vi "__AttrMap-SetValue2.vi"(8 "error in (no error)":errorcluster, 9 "Key":string, 10 "Value":variant, 11 "AttrMap in":T1) -> (0 "error out":errorcluster, 3 "AttrMap out":T1)   [LabVIEW 2019]
uses:
  Typedef/Def-AttrMap.ctl
  6e91e2cf-a420-477d-bf86-627245081caf.vi
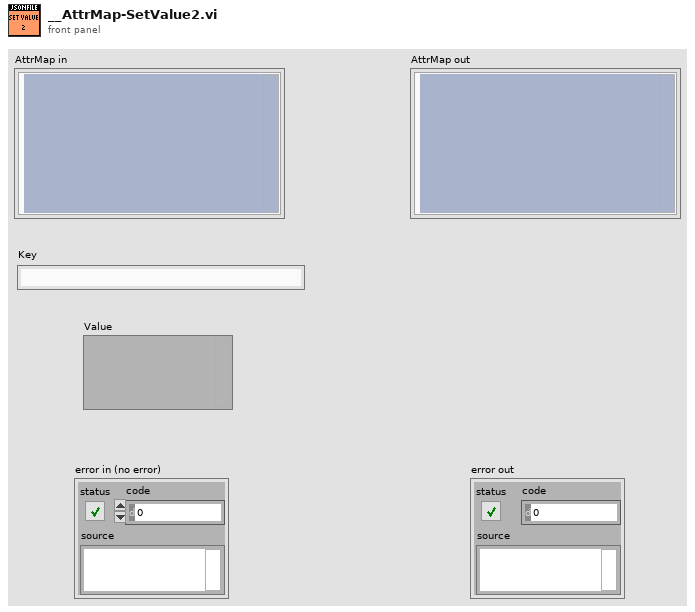
[diagram p1: front panel]
types:
  T1 = typedef "Def-AttrMap.ctl" = cluster{"Map":variant}
  T2 = typedef "Def-NameMap.ctl" = variant[]
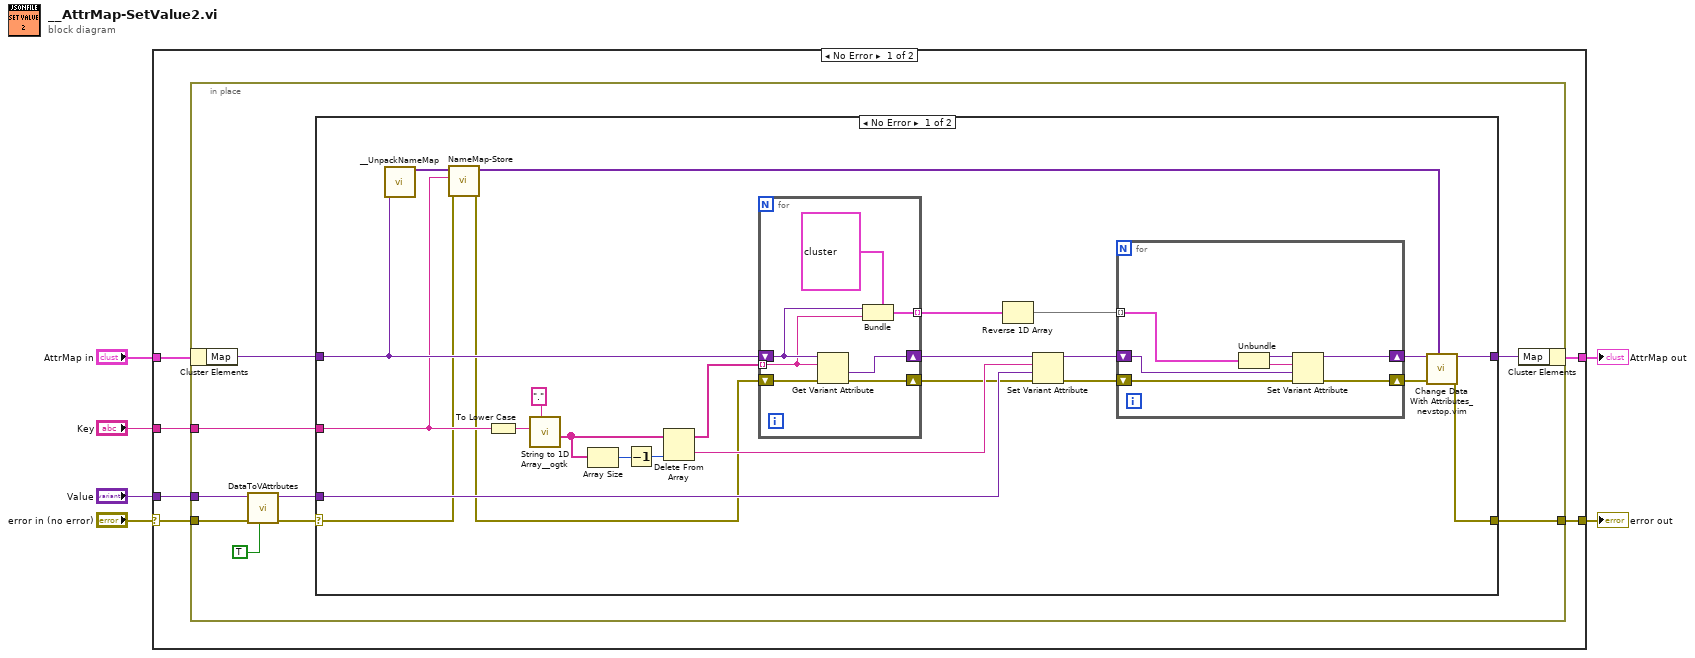
[diagram p0: block diagram]
diagram:
  n1 = case shown="No Error" "error in (no error)" {
    selector: "error in (no error)" -> [w11 w62]
    tunnel: [w12 w62] -> w6
    tunnel: "Key" -> [w10 _]
    tunnel: "Value" -> [w9 _]
    tunnel: "AttrMap in" -> [w8 w63]
    tunnel: [w7 w63] -> w1
    frame No Error {
      n2 = in-place {
        in-place-border: [w21] -> w12
        in-place-border: w11 -> [w15]
        in-place-border: w10 -> [w16]
        in-place-border: w9 -> [w18]
        n3 = in-place-cluster #1(w8) -> ("Map"=w19:variant)
        n4 = call "DataToVAttrbutes.vi"("to lowercase?(T)"=TRUE, "error in (no error)"=w15, "data"=w18) -> ("error out"=w13:errorcluster, "VAttributes"=w17:variant)  [unwired: 7 in]
        n5 = case shown="No Error" w13 {
          selector: w13 -> [w24 w60]
          tunnel: [w45 w60] -> w21
          tunnel: [w44 w61] -> w20
          tunnel: w19 -> [w42 w61]
          tunnel: w17 -> [w31 _]
          tunnel: w16 -> [w28 _]
          frame No Error {
            n6 = call "__UnpackNameMap.vi"("Map"=w42) -> ("NameMap"=w30:T2)  [unwired: 10 in]
            n7 = call "NameMap-Store.vi"("error in (no error)"=w24, "name"=w28, "NameMap in"=w30) -> ("error out"=w23:errorcluster, "NameMap out"=w29:T2)  [unwired: 7 in]
            n8 = To Lower Case(string=w28) -> (all lower case string=w40:string)
            n9 = call <userlib>:"String to 1D Array__ogtk.vi"("delimiter (Tab)"=".", "string"=w40) -> ("Array of Strings"=w37:string[])  [unwired: 9 in]
            n10 = Array Size(array=w37) -> (size(s)=w41:i32)
            n11 = Decrement(x=w41) -> (x-1=w32:i32)
            n12 = Delete From Array(array=w37, index=w32) -> (deleted portion=w38:string, array with subset deleted=w36:string[])  [unwired: 1 in]
            n13 = for {
              tunnel: w36 -> [w58] mode=indexing
              shift-right: [w57] -> w39
              shift-left: w42 -> [w59]
              tunnel: [w55] -> w35 mode=indexing
              shift-right: [w54] -> w25
              shift-left: w23 -> [w53]
              n14 = Get Variant Attribute(Variant=w59, name=w58, error in=w53) -> (value=w57:variant, error out=w54:errorcluster)  [unwired: 1 in, 2 out]
              n15 = Bundle(cluster=cluster{"Parent":variant, "Name":string} {"Parent"=variant, "Name"=""}, "Parent"=w59, "Name"=w58) -> (w55:cluster{"Parent":variant, "Name":string})
            }
            n16 = Reverse 1D Array(array=w35) -> (reversed array=w22:cluster{"Parent":variant, "Name":string}[])
            n17 = Set Variant Attribute(Variant=w39, name=w38, value=w31, error in=w25) -> (Variant out=w34:variant, error out=w27:errorcluster)  [unwired: 1 out]
            n18 = for {
              tunnel: w22 -> [w52] mode=indexing
              shift-right: [w51] -> w33
              shift-left: w34 -> [w48]
              shift-right: [w46] -> w26
              shift-left: w27 -> [w47]
              n19 = Unbundle(w52) -> ("Parent"=w50:variant, "Name"=w49:string)
              n20 = Set Variant Attribute(Variant=w50, name=w49, value=w48, error in=w47) -> (Variant out=w51:variant, error out=w46:errorcluster)  [unwired: 1 out]
            }
            n21 = call "Change Data With Attributes_nevstop.vim"("Data"=w29, "error in (no error)"=w26, "Variant in"=w33) -> ("error out"=w45:errorcluster, "Variant out"=w44:variant)  [unwired: 7 in]
          }
          frame Error {
          }
        }
        n22 = in-place-cluster #1("Map"=w20) -> (w7:T1)
      }
    }
    frame Error {
    }
  }
  "error out" <- w6
  "AttrMap out" <- w1
